vi "FTW-JSON-Destroy.vi"(0 "JSON Object":refnum<class "FTW-JSON.lvclass">, 11 "error in":errorcluster) -> (15 "error out":errorcluster)   [LabVIEW 2013, in "FTW-JSON.lvclass"]
uses:
  FTW-JSON.lvclass
  FTW-JSON.lvclass/FTW-JSON.ctl
panel:
  # "Inputs"
  # "Outputs"
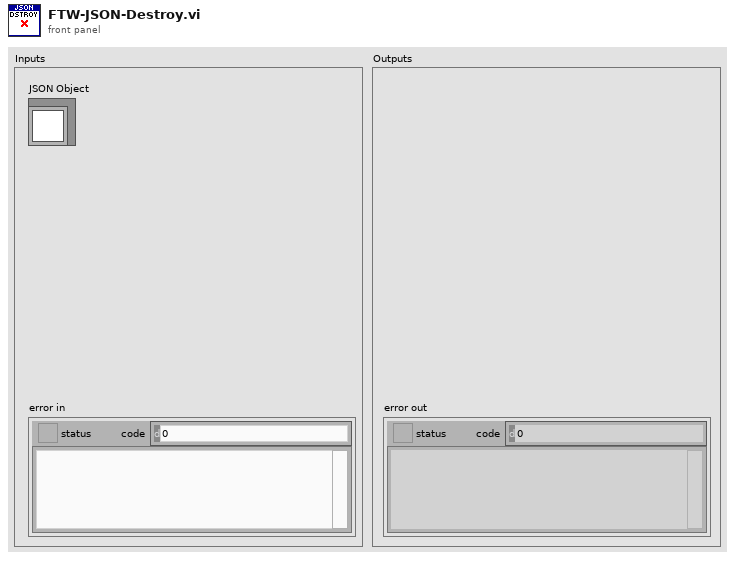
[diagram p1: front panel]
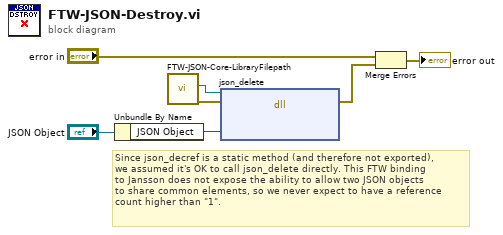
[diagram p0: block diagram]
diagram:
  # "Since json_decref is a static method (and therefore not exported),\nwe assumed it's OK to call json_delete directly. This FTW binding\nto Jansson does not expose the ability to allow two JSON objects\nto share common elements, so we never expect to have a reference\ncount higher than \"1\"."
  n1 = Unbundle By Name("JSON Object") -> ("JSON Object"=w4:i64)
  n2 = call "FTW-JSON-Core-LibraryFilepath.vi"() -> ("error out"=w7:errorcluster, "JSON Library Filepath"=w6:path)  [unwired: 10 in]
  n3 = dll-call lib="?" fn="json_delete"(path in=w6, error in=w7, "JSON Object Pointer"=w4) -> (error out=w2:errorcluster)  [unwired: 3 in, 1 out]
  n4 = Merge Errors("error in", w2) -> (→"error out":errorcluster)
